vi "Get Joint Angles.vi"(8 "error in (no error)":errorcluster, 11 "GripsMaster in":refnum<class "GripsMaster.lvclass">) -> (0 "error out":errorcluster, 1 "simulator_angles":dbl[](array[numeric]), 2 "joint_angles":dbl[](array[numeric]), 3 "GripsMaster out":refnum<class "GripsMaster.lvclass">)   [LabVIEW 2011, in "GripsMaster.lvclass"]
uses:
  GripsMaster.lvclass
  GripsMaster.lvclass/GripsMaster.ctl
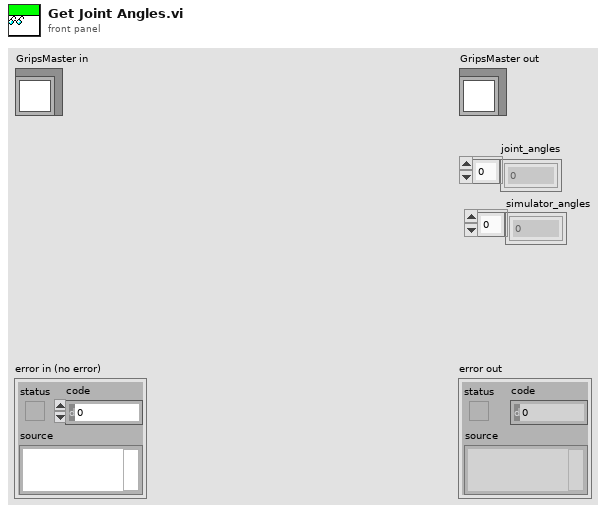
[diagram p1: front panel]
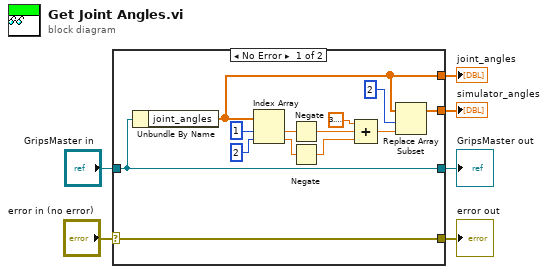
[diagram p0: block diagram]
diagram:
  n1 = case shown="No Error" "error in (no error)" {
    selector: "error in (no error)" -> [w19 w20]
    tunnel: [w19 w20] -> w5
    tunnel: [w18 w21] -> w3
    tunnel: "GripsMaster in" -> [w18 w21]
    tunnel: [w15 _] -> w2
    tunnel: [w7 _] -> w1
    frame No Error {
      n2 = Unbundle By Name(w18) -> ("joint_angles"=w15:dbl[])
      n3 = Index Array(array=w15, index #1=1 ("index"), index #2=2 ("index")) -> (element #1=w12:dbl, element #2=w11:dbl)
      n4 = Negate(x=w12) -> (-x=w10:dbl)
      n5 = Negate(x=w11) -> (-x=w9:dbl)
      n6 = Compound Arithmetic op=ADD(3.141592653589793, w10, w9) -> (w13:dbl)
      n7 = Replace Array Subset(array=w15, new element=w13, index=2) -> (w7:dbl[])
    }
    frame Error {
    }
  }
  "error out" <- w5
  "GripsMaster out" <- w3
  "joint_angles" <- w2
  "simulator_angles" <- w1
